vi "CircleFinderAI.vi"(0 "Image Type":T8 items=["Grayscale (U8)", "Grayscale (I16)", "Grayscale (SGL)", "Complex (CSG)", "RGB (U32)", "HSL (U32)", "RGB (U64)", "Grayscale (U16)"], 1 "Session In":T2="cam1", 5 "Curve Parameters":T7={"Extraction Mode"=0, "Edge Threshold"=100, "Edge Filter Size"=1, "Min Length"=10, "Row Search Step Size"=10, "Col Search Step Size"=100, "Max Endpoint Gap"=100, "Closed"=FALSE, "Subpixel"=FALSE} {"Max Endpoint Gap" min=0; "Col Search Step Size" min=1 max=255 step=1; "Row Search Step Size" min=1 max=255 step=1; "Min Length" min=0; "Edge Filter Size" items=["Fine", "Normal", "Controur Tracing"]; "Edge Threshold" min=1 max=65535 step=1; "Extraction Mode" items=["Normal", "Uniform Regions"]}, 9 "Circle Descriptor":cluster{"Min Radius":dbl, "Max Radius":dbl}={"Min Radius"=25.0, "Max Radius"=45.0}, 11 "error in (no error)":errorcluster, 12 "Image Name":string="name1") -> (3 "Image":T3(plugin-control), 4 "NumCirclesFound":i32, 6 "Circle0":T1, 10 "AllCircles":T6(array[cluster]) {"Position"."Y" format="%.2f"; "Position"."X" format="%.2f"}, 15 "error out":errorcluster)   [LabVIEW 2019]
uses:
  <vilib>/vision/Pattern Matching.llb/IMAQ Curve Parameters.ctl
  <vilib>/vision/Shape Detection.llb/ShapeDetectionMatchOptions.ctl
  <vilib>/vision/Pattern Matching.llb/IMAQ Match Range Setting.ctl
  <vilib>/userDefined/High Color/IMAQdx.ctl
  <vilib>/vision/driver/NI_Vision_Acquisition_Software.lvlib
  <vilib>/vision/NI_Vision_Development_Module.lvlib
panel:
  out "Circle0Params":string
  in  "Match Options":T4 {"Range Settings"."Match Constraints" items=["Rotation Angle (degrees)", "Scale Factor (%)", "Occlusion (%)"]}
  # "Range"
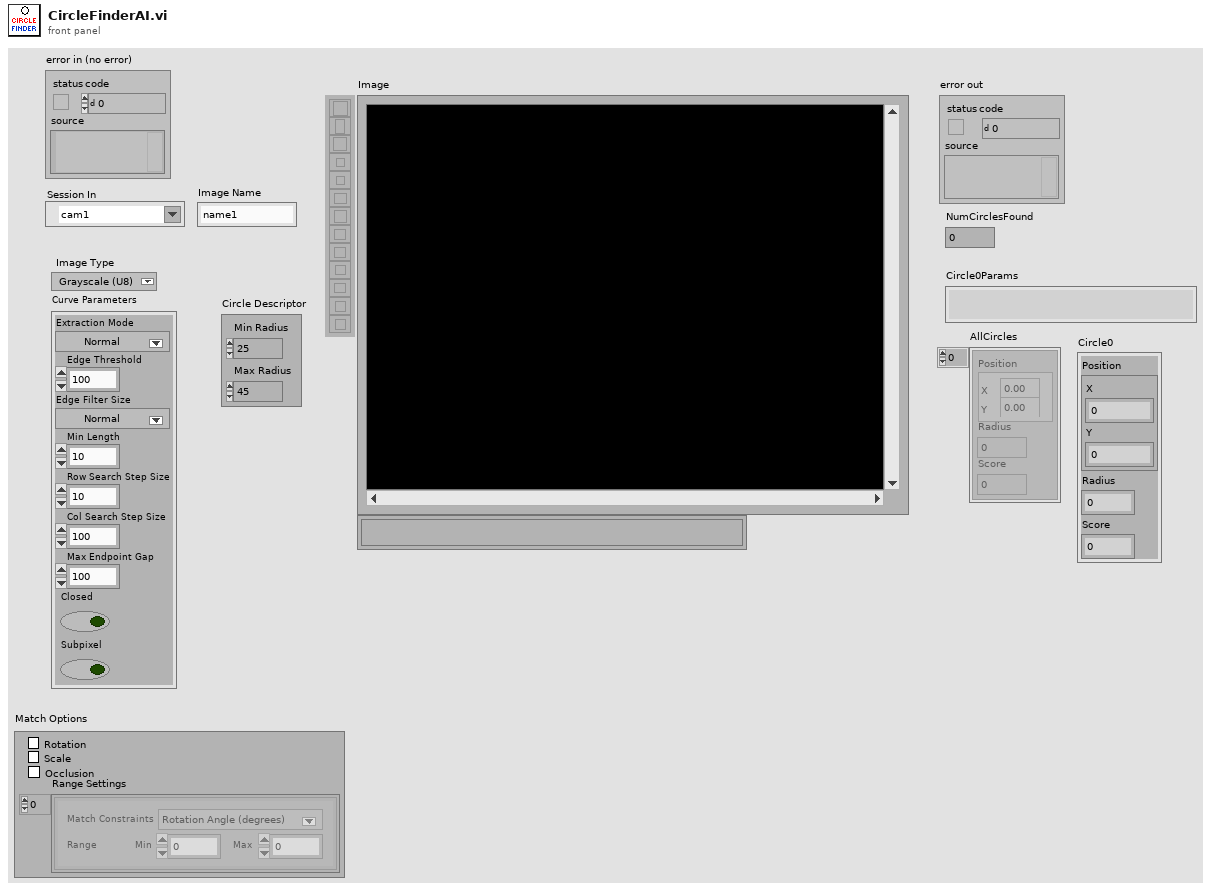
[diagram p1: front panel]
types:
  T1 = cluster{"Position":cluster{"X":sgl, "Y":sgl}, "Radius":dbl, "Score":dbl}
  T2 = typedef "IMAQdx.ctl" = refnum<k21>
  T3 = typedef "IMAQ Image.ctl" = refnum<image>
  T4 = typedef "ShapeDetectionMatchOptions.ctl" = cluster{"Rotation":bool, "Scale":bool, "Occlusion":bool, "Range Settings":T5[]}
  T5 = typedef "IMAQ Match Range Setting.ctl" = cluster{"Match Constraints":u32, "Min":dbl, "Max":dbl}
  T6 = cluster{"Position":cluster{"X":sgl, "Y":sgl}, "Radius":dbl, "Score":dbl}[]
  T7 = typedef "IMAQ Curve Parameters.ctl" = cluster{"Extraction Mode":u32, "Edge Threshold":i32, "Edge Filter Size":u32, "Min Length":i32, "Row Search Step Size":i32, "Col Search Step Size":i32, "Max Endpoint Gap":i32, "Closed":bool, "Subpixel":bool}
  T8 = typedef "Image Type" = u32
  T9 = typedef "IMAQ Circle" = cluster{"Center X":i32, "Center Y":i32, "Inner Radius":i32, "Outer Radius":i32, "Start Angle":dbl, "End Angle":dbl}
  T10 = cluster{"Circles[0]":cluster{"Position":cluster{"X":sgl, "Y":sgl}, "Radius":dbl, "Score":dbl}, "Circles[1]":cluster{"Position":cluster{"X":sgl, "Y":sgl}, "Radius":dbl, "Score":dbl}, "Circles[2]":cluster{"Position":cluster{"X":sgl, "Y":sgl}, "Radius":dbl, "Score":dbl}, "Circles[3]":cluster{"Position":cluster{"X":sgl, "Y":sgl}, "Radius":dbl, "Score":dbl}, "Circles[4]":cluster{"Position":cluster{"X":sgl, "Y":sgl}, "Radius":dbl, "Score":dbl}, "Circles[5]":cluster{"Position":cluster{"X":sgl, "Y":sgl}, "Radius":dbl, "Score":dbl}, "Circles[6]":cluster{"Position":cluster{"X":sgl, "Y":sgl}, "Radius":dbl, "Score":dbl}, "Circles[7]":cluster{"Position":cluster{"X":sgl, "Y":sgl}, "Radius":dbl, "Score":dbl}, "Circles[8]":cluster{"Position":cluster{"X":sgl, "Y":sgl}, "Radius":dbl, "Score":dbl}}
  T11 = typedef "ROI Descriptor" = cluster{"Global Rectangle":i32[], "Contours":cluster{"ID":enum32{"External", "Internal"}, "Type":u32, "Coordinates":i32[]}[]}
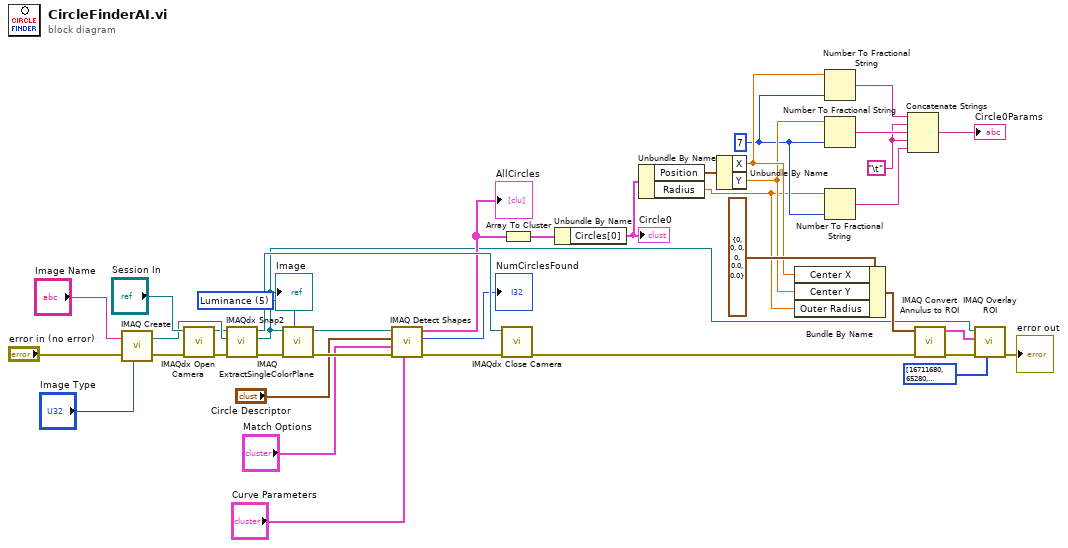
[diagram p0: block diagram]
diagram:
  w1 = 5 items=["Red", "Green", "Blue", "Hue", "Saturation", "Luminance", "Value", "Intensity"] ("Color Plane")
  w7 = "\t"
  w6 = i16 7 ("precision (6)")
  n1 = call "IMAQ Create"("Image Name"="Image Name", "Image Type"="Image Type", "error in (no error)"="error in (no error)") -> ("New Image"=w36:T3, "error out"=w33:errorcluster)  [unwired: 2 in]
  n2 = call <vilib>:"IMAQdx Open Camera.vi"("error in"=w33, "Session In"="Session In") -> ("error out"=w37:errorcluster, "Session Out"=w35:T2)  [unwired: 8 in]
  n3 = call <vilib>:"IMAQdx Snap2.vi"("error in"=w37, "Image In"=w36, "Session In"=w35) -> ("error out"=w29:errorcluster, "Image Out"=w2:T3, "Session Out"=w34:T2)  [unwired: 6 in]
  "Image" <- w2
  n4 = call "IMAQ ExtractSingleColorPlane"("Color Plane"=w1, "error in (no error)"=w29, "Image Src"=w2) -> ("error out"=w28:errorcluster, "Image Dst Out"=w24:T3)  [unwired: 1 in, 6 out]
  n5 = call-poly "IMAQ Detect Shapes"("Curve Parameters"="Curve Parameters", "error in (no error)"=w28, "Match Options"="Match Options", "Circle Descriptor"="Circle Descriptor", "Image"=w24) -> ("error out"=w31:errorcluster, "Number of Matches Returned"=→"NumCirclesFound":i32, "Circles"=w20:T6)  [unwired: 2 in, 2 out]
  "AllCircles" <- w20
  n6 = call <vilib>:"IMAQdx Close Camera.vi"("error in"=w31, "Session In"=w34) -> ("error out"=w17:errorcluster)  [unwired: 9 in]
  n7 = Array To Cluster(array=w20) -> (cluster=w19:T10)
  n8 = Unbundle By Name(w19) -> ("Circles[0]"=w18:T1)
  "Circle0" <- w18
  n9 = Unbundle By Name(w18) -> ("Position"=w21:cluster{"X":sgl, "Y":sgl}, "Radius"=w5:dbl)
  n10 = Unbundle By Name(w21) -> ("X"=w12:sgl, "Y"=w11:sgl)
  n11 = Bundle By Name(cluster=T9 {"Center X"=0, "Center Y"=0, "Inner Radius"=0, "Outer Radius"=0, "Start Angle"=0.0, "End Angle"=0.0} ("Annulus"), "Center X"=w12, "Center Y"=w11, "Outer Radius"=w5) -> (w23:T9)
  n12 = Number To Fractional String(number=w12, precision (6)=w6) -> (F-format string=w10:string)  [unwired: 2 in]
  n13 = Number To Fractional String(number=w11, precision (6)=w6) -> (F-format string=w9:string)  [unwired: 2 in]
  n14 = Number To Fractional String(number=w5, precision (6)=w6) -> (F-format string=w4:string)  [unwired: 2 in]
  n15 = Concatenate Strings(w10, w7, w9, w7, w4) -> (→"Circle0Params":string)
  n16 = call "IMAQ Convert Annulus to ROI"("error in (no error)"=w17, "Annulus"=w23) -> ("error out"=w15:errorcluster, "ROI Descriptor"=w16:T11)  [unwired: 7 in]
  n17 = call "IMAQ Overlay ROI"("Colors (Green)"=u32[] [16711680, 65280, 2626303], "error in (no error)"=w15, "ROI Descriptor"=w16, "Image"=w2) -> ("error out"=→"error out":errorcluster)  [unwired: 6 in, 1 out]
